vi "A_8.vi"() -> ()   [LabVIEW 2020]
uses:
  <vilib>/numeric/Random Number (Range) DBL.vi
panel:
  in  "stop":bool
  out "Plane coordinates":string
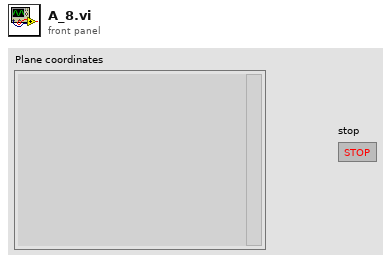
[diagram p1: front panel]
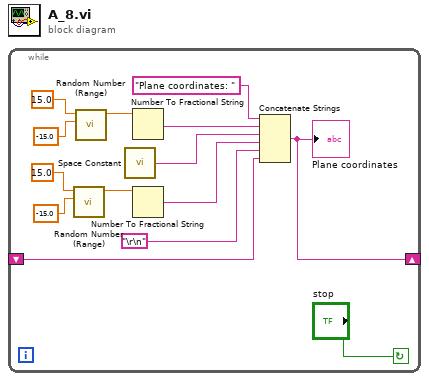
[diagram p0: block diagram]
diagram:
  n1 = while {
    shift-right: [w2] -> _
    shift-left: _ -> [w1]
    stop <- "stop" continue-if-true
    n2 = call-poly <vilib>:"Random Number (Range).vi"("lower bound (0)"=-15.0, "upper bound (100)"=15.0) -> ("number"=w7:dbl)  [unwired: 9 in]
    n3 = call-poly <vilib>:"Random Number (Range).vi"("lower bound (0)"=-15.0, "upper bound (100)"=15.0) -> ("number"=w8:dbl)  [unwired: 9 in]
    n4 = call <vilib>:"Space Constant.vi"() -> ("String"=w6:string)
    n5 = Number To Fractional String(number=w8) -> (F-format string=w5:string)  [unwired: 3 in]
    n6 = Number To Fractional String(number=w7) -> (F-format string=w4:string)  [unwired: 3 in]
    n7 = Concatenate Strings("Plane coordinates: ", w5, w6, w4, "\r\n", w1) -> (w2:string)
    "Plane coordinates" <- w2
  }
